vi "Result_Test.vi"(8 "error in (no error)":errorcluster caption="entrée d'erreur (pas d'erreur)", 11 "Get_Voltage en entrée":refnum<class "Zigbee_Write_Msg.lvclass">) -> (0 "error out":errorcluster caption="sortie d'erreur", 3 "Get_Voltage en sortie":refnum<class "Zigbee_Write_Msg.lvclass">)   [LabVIEW 2020, in "Library Test.lvlib" / "Zigbee_Write_Msg.lvclass"]
uses:
  Zigbee_Write_Msg.lvclass
  C:/Users/ngarcin/OneDrive - Altyor/Standard TB/Class/Test/Test (Default)/Test (Default).lvclass
  Zigbee_Send_Command_UART/Zigbee_Send_Command_UART.lvclass
  Zigbee_Write_Msg.lvclass/Zigbee_Write_Msg.ctl
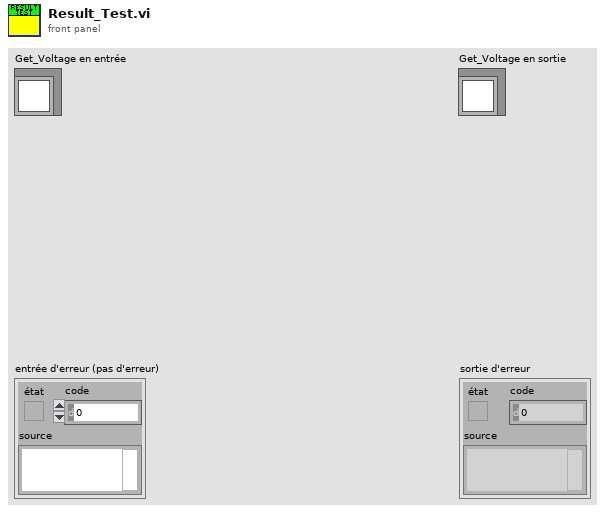
[diagram p1: front panel]
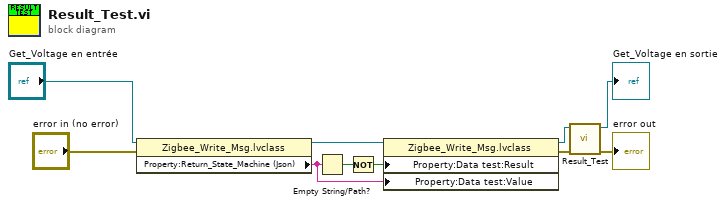
[diagram p0: block diagram]
diagram:
  n1 = property class="Zigbee_Write_Msg.lvclass"(reference="Get_Voltage en entrée", error in="error in (no error)") -> (reference out=w8:refnum<class "Zigbee_Write_Msg.lvclass">, "Property:Return_State_Machine (Json)"=w5:string)  [unwired: 1 out]
  n2 = Empty String/Path?(string/path=w5) -> (empty?=w7:bool)
  n3 = Not(x=w7) -> (.not. x?=w6:bool)
  n4 = property class="Zigbee_Write_Msg.lvclass"(reference=w8, "Property:Data test:Result"=w6, "Property:Data test:Value"=w5) -> (reference out=w2:refnum<class "Zigbee_Write_Msg.lvclass">, error out=w1:errorcluster)  [unwired: 1 in]
  n5 = call-parent "Result_Test.vi"("error in (no error)"=w1, "Get_Voltage en entrée"=w2) -> ("error out"=→"error out":errorcluster, "Get_Voltage en sortie"=→"Get_Voltage en sortie":refnum<class "Zigbee_Write_Msg.lvclass">)  [unwired: 8 in]
